vi "Memory.Pointer.Coerce Subset.vi"(7 "source vi name":string, 8 "error in (no error)":errorcluster, 9 "length (-1: rest)":i64=-1 format="%d bytes", 10 "offset (0)":u64 format="%d bytes", 11 "pointer in":refnum<class "Memory.Pointer.lvclass">) -> (0 "error out":errorcluster, 1 "length":u64 format="%d bytes", 2 "offset":u64 format="%d bytes", 3 "pointer out":refnum<class "Memory.Pointer.lvclass">)   [LabVIEW 2016, in "Memory.lvlib" / "Memory.Pointer.lvclass"]
uses:
  Memory.Pointer.lvclass
  Memory.Pointer.Errors.Out of Bounds.vi
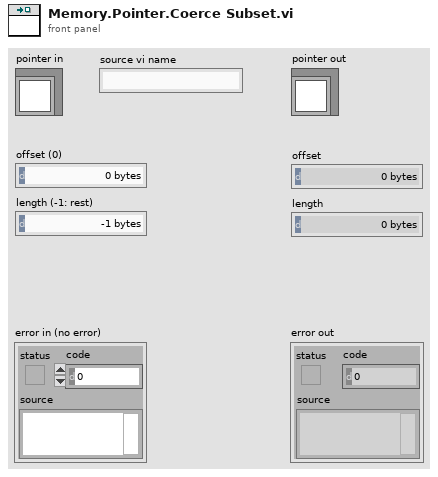
[diagram p1: front panel]
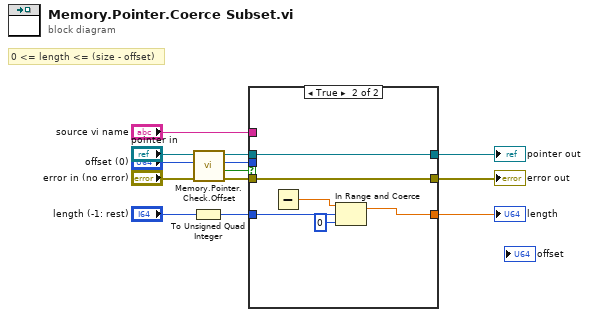
[diagram p0: block diagram]
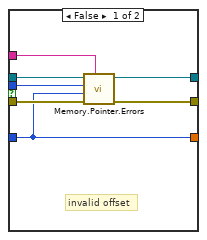
[diagram p2: hidden frame]
diagram:
  # "0 <= length <= (size - offset)"
  n1 = To Unsigned Quad Integer(1:"length (-1: rest)") -> (0:w10:u64)
  n2 = call "Memory.Pointer.Check.Offset.vi"("offset in"="offset (0)", "Pointer in"="pointer in") -> ("valid offset?"=w4:bool, "offset out"=w5:u64, "Pointer out"=w7:refnum<class "Memory.Pointer.lvclass">)  [unwired: 7 in]
  n3 = case shown="True" w4 {
    tunnel: w10 -> [w13 w24]
    tunnel: [w13 w22] -> w8
    tunnel: w7 -> [w19 w21]
    tunnel: [w18 w21] -> w6
    tunnel: w5 -> [w15 _]
    tunnel: "error in (no error)" -> [w17 w20]
    tunnel: [w16 w20] -> w2
    tunnel: "source vi name" -> [w14 _]
    frame False {
      # "invalid offset"
      n4 = call-poly "Memory.Pointer.Errors.vi"("source vi name"=w14, "error in (no error)"=w17, "length"=w13, "offset"=w15, "pointer in"=w19) -> ("error out"=w16:errorcluster, "pointer out"=w18:refnum<class "Memory.Pointer.lvclass">)  [unwired: 5 in]
    }
    frame True {
      n5 = Subtract() -> (x-y=w23:dbl)  [unwired: 2 in]
      n6 = In Range and Coerce(upper limit=w23, x=w24, lower limit=u64 0) -> (coerced(x)=w22:dbl)  [unwired: 1 out]
    }
  }
  "error out" <- w2
  "pointer out" <- w6
  "length" <- w8
